vi "Diff_Drive_Simulated_Hardware.vi"(7 "body_mass(kg)":dbl, 8 "delta_t":dbl, 9 "c(friction)":dbl, 10 "u_right(N)":dbl, 11 "u_left(N)":dbl) -> (0 "v_angular":dbl, 1 "x_angular":dbl, 2 "a_linear":dbl, 3 "v_linear":dbl, 4 "a_angular":dbl)   [LabVIEW 2019]
panel:
  in  "b_length":dbl
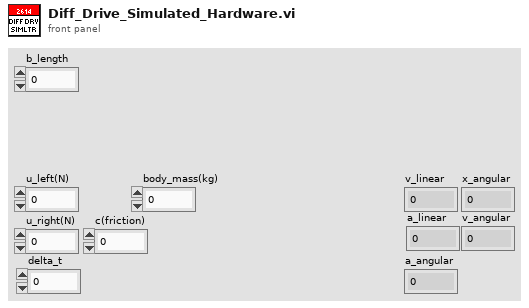
[diagram p1: front panel]
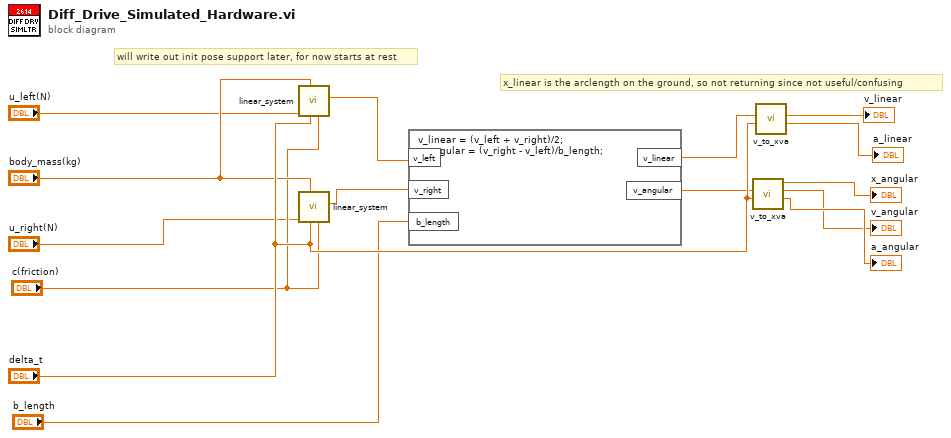
[diagram p0: block diagram]
diagram:
  # "x_linear is the arclength on the ground, so not returning since not useful/confusing"
  # "will write out init pose support later, for now starts at rest"
  n1 = call "linear_system.vi"("c(friction)"="c(friction)", "delta_t"="delta_t", "m(mass)"="body_mass(kg)", "u_in(input force)"="u_left(N)") -> ("v_out"=w6:dbl)  [unwired: 5 in, 2 out]
  n2 = call "linear_system.vi"("c(friction)"="c(friction)", "delta_t"="delta_t", "m(mass)"="body_mass(kg)", "u_in(input force)"="u_right(N)") -> ("v_out"=w7:dbl)  [unwired: 5 in, 2 out]
  n3 = formula code="v_linear = (v_left + v_right)/2;\nv_angular = (v_right - v_left)/b_length;"("v_left"=w6, "v_right"=w7, "b_length"="b_length") -> ("v_angular"=w9:dbl, "v_linear"=w8:dbl)
  n4 = call "v_to_xva.vi"("dt"="delta_t", "v"=w9) -> ("a_out"=→"a_angular":dbl, "v_out"=→"v_angular":dbl, "x_out"=→"x_angular":dbl)  [unwired: 7 in]
  n5 = call "v_to_xva.vi"("dt"="delta_t", "v"=w8) -> ("a_out"=→"a_linear":dbl, "v_out"=→"v_linear":dbl)  [unwired: 7 in, 1 out]
